vi "区域判断.vi"(4 "压力数组":dbl[](array[numeric]), 5 "位移数组":dbl[](array[numeric]), 6 "区域最大压力":dbl, 7 "区域最小压力":dbl, 8 "区域最大位移":dbl, 9 "区域最小位移":dbl) -> (0 "数值 2":dbl, 1 "数值":dbl, 3 "区域监控合格":bool)   [LabVIEW 2013]
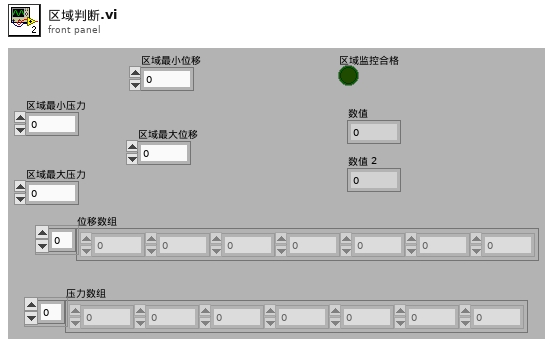
[diagram p1: front panel]
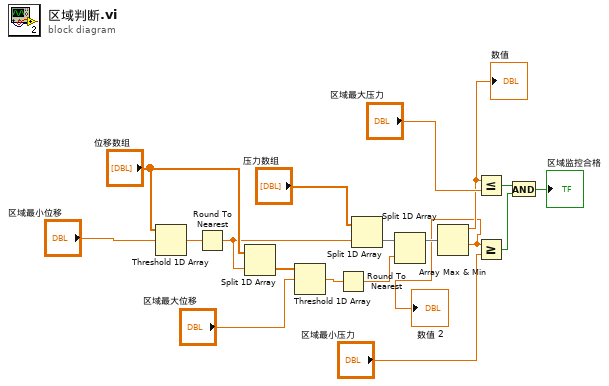
[diagram p0: block diagram]
diagram:
  n1 = Threshold 1D Array(2:"区域最小位移", 3:"位移数组") -> (0:w16:dbl)  [unwired: 1 in]
  n2 = Round To Nearest(number=w16) -> (nearest integer value=w12:dbl)
  n3 = Split 1D Array(array="位移数组", index=w12) -> (second subarray=w13:dbl[])  [unwired: 1 out]
  n4 = Threshold 1D Array(2:"区域最大位移", 3:w13) -> (0:w1:dbl)  [unwired: 1 in]
  n5 = Round To Nearest ("最近数取整")(number=w1) -> (nearest integer value=w10:dbl)
  n6 = Split 1D Array(array="压力数组", index=w12) -> (second subarray=w11:dbl[])  [unwired: 1 out]
  n7 = Split 1D Array(array=w11, index=w10) -> (first subarray=w9:dbl[])  [unwired: 1 out]
  n8 = Array Max & Min(array=w9) -> (max value=w3:dbl, min value=w2:dbl)  [unwired: 2 out]
  "数值" <- w3
  "数值 2" <- w2
  n9 = Less Or Equal?(x=w3, y="区域最大压力") -> (x <= y?=w6:bool)
  n10 = Greater Or Equal?(x=w2, y="区域最小压力") -> (x >= y?=w5:bool)
  n11 = And(x=w6, y=w5) -> (x .and. y?=→"区域监控合格":bool)
